vi "Initialize.vi"(5 "timeout, ms (300)":u32=300, 6 "stop bits (1.0)":u16(ring)=10 items=["1.0"=10, "2.0"=20], 7 "address (1)":u8=1, 8 "error in (no error)":errorcluster, 9 "parity (none)":enum16{"None", "Odd", "Even", "Mark", "Space"}(ring), 10 "baud rate (19200)":u32(ring)=19200 items=["1200"=1200, "2400"=2400, "4800"=4800, "9600"=9600, "19200"=19200, "38400"=38400, "57600"=57600, "115200"=115200], 11 "port":refnum<visa-resource-name>) -> (0 "error out":errorcluster, 3 "HFP Gen out":refnum<class "PL HFP Generator.lvclass">)   [LabVIEW 2015, in "PL HFP Generator.lvclass"]
doc: "Initializes connection to device using specified settings."
uses:
  PL HFP Generator.lvclass
  <vilib>/plasmapper/PL Modbus Client/PL Modbus Client.lvclass
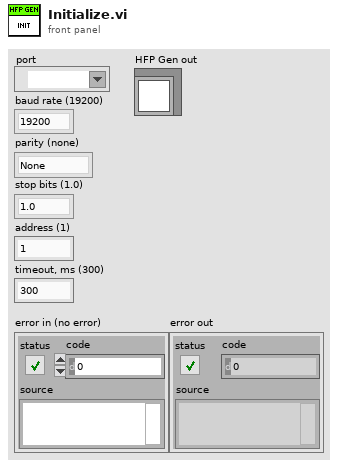
[diagram p1: front panel]
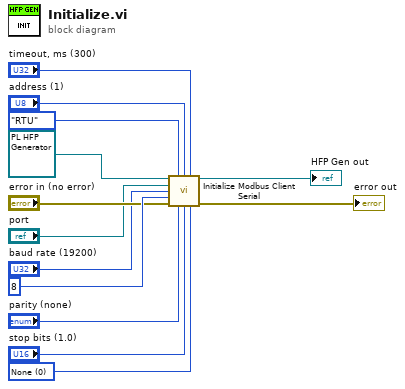
[diagram p0: block diagram]
diagram:
  w8 = u16 0 items=["None", "XON/XOFF", "RTS/CTS", "XON/XOFF & RTS/CTS", "DTR/DSR", "XON/XOFF & DTR/DSR"] ("flow control (none)")
  n1 = call <vilib>:"Initialize Modbus Client Serial.vi"("MODBUS in"=refnum<class "PL HFP Generator.lvclass"> refnum ("Eltochpribor RRG.lvclass"), "protocol (RTU)"=enum16{"RTU", "ASCII", "TCP"}."RTU", "station address (1)"="address (1)", "timeout, ms (300)"="timeout, ms (300)", "port"="port", "baud rate (9600)"="baud rate (19200)", "data bits (8)"=u16 8, "error in (no error)"="error in (no error)", "parity (even)"="parity (none)", "stop bits (1.0)"="stop bits (1.0)", "flow control (none)"=w8) -> ("MODBUS out"=→"HFP Gen out":refnum<class "PL HFP Generator.lvclass">, "error out"=→"error out":errorcluster)  [unwired: 3 in]
